vi "Decimate (single shot, DBL).vi"(9 "averaging":bool, 10 "decimating factor":i32=1, 11 "X":dbl[](array[numeric])) -> (0 "error":i32, 3 "Decimated Array":dbl[](array[numeric]))   [LabVIEW 2017, in "NI_AALPro.lvlib"]
doc: "Decimates the input sequence <B>X</B> by the <B>decimating factor</B> and the <B>averaging</B> Boolean control. Wire data to the <B>X</B> input to determine the polymorphic instance to use or manually select the instance."
uses:
  NI_AALPro.lvlib
  lvanlys.dll
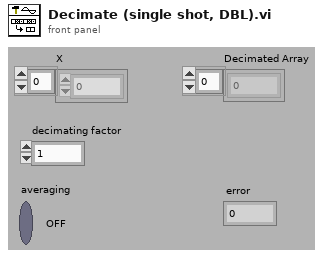
[diagram p1: front panel]
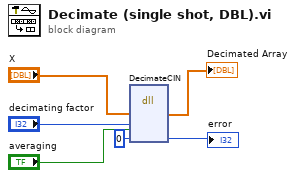
[diagram p0: block diagram]
diagram:
  n1 = dll-call lib="C:/Program Files/National Instruments/LabVIEW 2017/resource/lvanlys.*" fn="DecimateCIN"("X"="X", "decimating factor"="decimating factor", "averaging"="averaging", "error"=0) -> ("X"=→"Decimated Array":dbl[], "error"=→"error":i32)  [unwired: 6 in, 2 out]
